vi "Model - Get TDMS Overhead.vi"(8 "error in (no error)":errorcluster, 11 "View Model":T2) -> (0 "error out":errorcluster, 1 "Use TDMS?":bool, 2 "FileSize":i32, 3 "View Model":T2, 4 "ChProps":T1={"AOM9"=[["Neutron LogN Power A", "Pump P2 MTTP", "Pump P3 MTTP", "Pump P4 MTTP", "Reserve AO1", "Reserve AO2"]], "AIM2"=[["Neutron LogN Power A", "Pump P2 MTTP", "Pump P3 MTTP", "Pump P4 MTTP", "Reserve AO1", "Reserve AO2"]], "DIM3"=[["Neutron LogN Power A", "Pump P2 MTTP", "Pump P3 MTTP", "Pump P4 MTTP", "Reserve AO1", "Reserve AO2"]], "DIM4"=[["Neutron LogN Power A", "Pump P2 MTTP", "Pump P3 MTTP", "Pump P4 MTTP", "Reserve AO1", "Reserve AO2"]], "DOM6"=[["Neutron LogN Power A", "Pump P2 MTTP", "Pump P3 MTTP", "Pump P4 MTTP", "Reserve AO1", "Reserve AO2"]], "DOM7"=[["Neutron LogN Power A", "Pump P2 MTTP", "Pump P3 MTTP", "Pump P4 MTTP", "Reserve AO1", "Reserve AO2"]]}, 5 "FileName":string)   [LabVIEW 2017]
doc: "Get actual value of TDMS Overhead cluster from DVR"
uses:
  Controls/View Model.ctl
  Controls/Shared Model.ctl
  Error Handler/Controls/Error Model.ctl
  Error Handler/Controls/Error Event.ctl
  Error Handler/Controls/Error Type.ctl
  Controller/Controls/Controller Model.ctl
  Controller/Controls/Controller Event.ctl
  Controller/Controls/Controller Command.ctl
  Controller/Controls/Controller Overhead.ctl
  Real-Time/RT Status.ctl
  Real-Time/RT Loop Status.ctl
  Controller/Controls/Controller NStream.ctl
  Controller/Controls/Controller Timer Data.ctl
  Controller/Controls/Controller DAQ Data.ctl
  TDMS Logger/Controls/TDMS Model.ctl
  TDMS Logger/Controls/TDMS Event.ctl
  TDMS Logger/Controls/TDMS Command.ctl
  TDMS Logger/Controls/TDMS Overhead.ctl
  TDMS Logger/Controls/TDMS ChanProperties.ctl
  TDMS Logger/Controls/TDMS DAQ Data.ctl
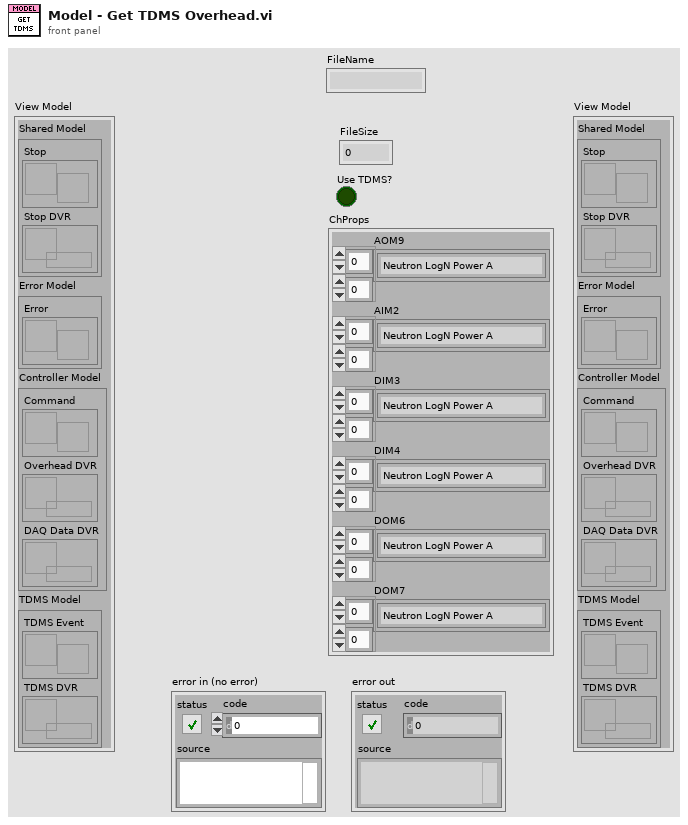
[diagram p1: front panel]
types:
  T1 = typedef "TDMS ChanProperties.ctl" = cluster{"AOM9":string[][], "AIM2":string[][], "DIM3":string[][], "DIM4":string[][], "DOM6":string[][], "DOM7":string[][]}
  T2 = typedef "View Model.ctl" = cluster{"Shared Model":T3, "Error Model":T4, "Controller Model":T5, "TDMS Model":T6}
  T3 = typedef "Shared Model.ctl" = cluster{"Stop":refnum<user-event>, "Stop DVR":refnum<data-value>}
  T4 = typedef "Error Model.ctl" = cluster{"Error":refnum<user-event>}
  T5 = typedef "Controller Model.ctl" = cluster{"Command":refnum<user-event>, "Overhead DVR":refnum<data-value>, "DAQ Data DVR":refnum<data-value>}
  T6 = typedef "TDMS Model.ctl" = cluster{"TDMS Event":refnum<user-event>, "TDMS DVR":refnum<data-value>}
  T7 = typedef "TDMS Overhead.ctl" = cluster{"FileName":string, "FileSize":i32, "Use TDMS?":bool, "Channel Properties":T1, "DAQ Data":T8}
  T8 = typedef "TDMS DAQ Data.ctl" = cluster{"AOM data":dbl[], "AIMV data":dbl[], "AIMC data":dbl[], "DOM data":dbl[], "DIM data":dbl[], "AOM timestamp":dbl, "AIMV timestamp":dbl, "AIMC timestamp":dbl, "DOM timestamp":dbl, "DIM timestamp":dbl}
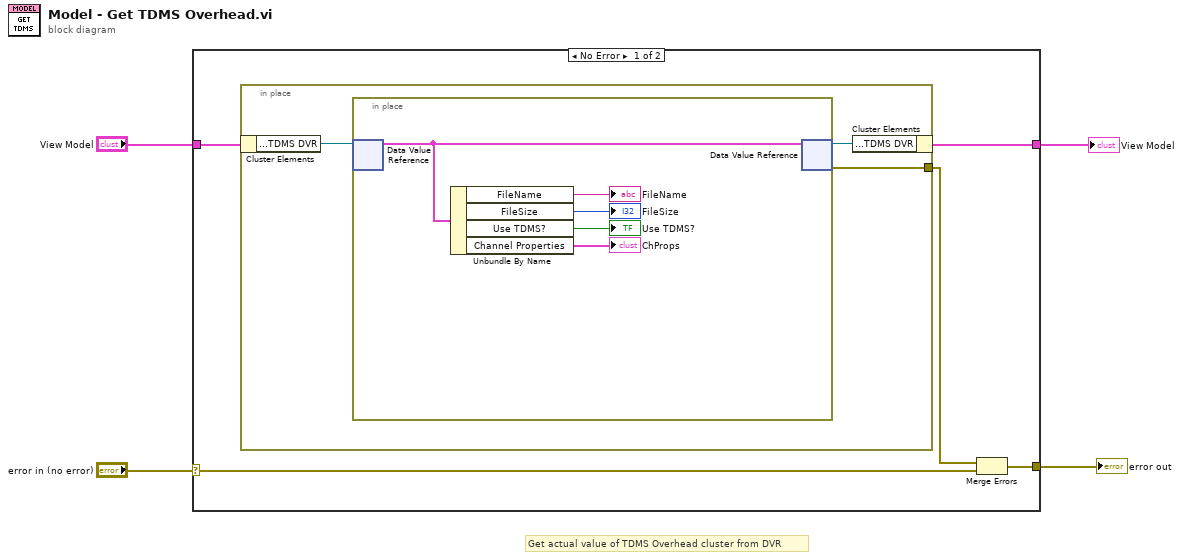
[diagram p0: block diagram]
diagram:
  # "Get actual value of TDMS Overhead cluster from DVR"
  n1 = case shown="No Error" "error in (no error)" {
    selector: "error in (no error)" -> [w6 w18]
    tunnel: "View Model" -> [w9 w19]
    tunnel: [w8 w19] -> w2
    tunnel: [w5 w18] -> w1
    frame No Error {
      n2 = in-place {
        in-place-border: [w10] -> w7
        n3 = in-place-cluster #1(w9) -> ("TDMS Model.TDMS DVR"=w12:refnum<data-value>)
        n4 = in-place {
          n5 = in-place-dvr #2(w12) -> (w17:T7)  [unwired: 1 out]
          n6 = Unbundle By Name(w17) -> ("FileName"=→"FileName":string, "FileSize"=→"FileSize":i32, "Use TDMS?"=→"Use TDMS?":bool, "Channel Properties"=→"ChProps":T1)
          n7 = in-place-dvr #2(w17) -> (w11:refnum<data-value>, w10:errorcluster)
        }
        n8 = in-place-cluster #1("TDMS Model.TDMS DVR"=w11) -> (w8:T2)
      }
      n9 = Merge Errors(w7, w6) -> (w5:errorcluster)
    }
    frame Error {
    }
  }
  "View Model" <- w2
  "error out" <- w1
